vi "PH_SHS_Analysis.check Cam Settings.vi"(0 "i ref in":refnum<vi>, 5 "error in":errorcluster) -> (14 "i ref out":refnum<vi>, 19 "error out":errorcluster)   [LabVIEW 2014, in "PH_SHS_Analysis.lvlib"]
doc: "This VI checks whether the current cam setting equels the cam settings of the calibration data file and indicates the result at the GUI."
uses:
  PH_SHS_Analysis.lvlib
  PH_Basics/PH_StatusHandler/PH_StatusHandler.Status.ctl
  PH_Basics/PH_Common/PH_Common.lvlib
  PH_Basics/PH_Img_BaseClass/PH_Img_BaseClass.lvlib
  PH_Basics/PH_StatusHandler/PH_StatusHandler.lvlib
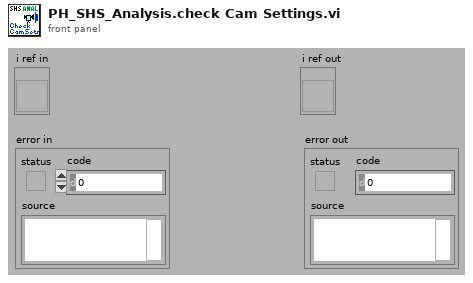
[diagram p1: front panel]
types:
  T1 = typedef "PH_StatusHandler.lvlib/PH_StatusHandler.Status.ctl" = i16
  T2 = typedef "PH_Img_BaseClass.lvlib/PH_Img_BaseClass.i attribute.ctl" = cluster{"GUI Refs":T3, "Timeout Image [ms]":i32, "Default Periodic Period [ms]":i32, "Camera":cluster{"Instancename":string, "Notifier":refnum<notifier>}, "Palette":T4, "Cam Settings":cluster{"Cam ID":string, "Gain":dbl, "Brightness":dbl, "Shutter":dbl, "Cam Info Failure":bool, "Mode":i32}}
  T3 = typedef "PH_Img_BaseClass.lvlib/PH_Img_BaseClass.GUI Refs.ctl" = cluster{"Timeout":refnum<vi>, "Image":refnum<vi>, "Palette":refnum<vi>, "Timeout Set":refnum<vi>}
  T4 = typedef "PH_Img_BaseClass.lvlib/PH_Img_BaseClass.Palette.ctl" = i32
  T5 = cluster{"Cam ID":string, "Gain":dbl, "Brightness":dbl, "Shutter":dbl, "Cam Info Failure":bool, "Mode":i32}
  T6 = typedef "PH_SHS_Analysis.lvlib/PH_SHS_Analysis.i attribute.ctl" = cluster{"GUI Refs":cluster{"Delete":refnum<vi>, "Global On":refnum<vi>, "Cam Source":refnum<vi>, "Calibration Data File":refnum<vi>, "Calibration status":refnum<vi>, "Show overlay":refnum<vi>, "SHS Device Config":refnum<vi>, "Result":refnum<vi>, "Consider Tilt":refnum<vi>, "Working Reference":refnum<vi>, "Remove Tilt":refnum<vi>, "Take Cali  Reference":refnum<vi>, "Publishing Data Status":refnum<vi>, "Calibration Data":refnum<vi>}, "Calibration":cluster{"Status":T1, "Data":T7, "File":path}, "Result":T12, "Image":T15, "SHS Device Config":T16, "Show Overlay":bool, "GradientZernikeMatrix":dbl[][], "Consider Tilt":bool, "Working Reference":T8, "Zernicke Service ID":i32, "PSDB Image":T15}
  T7 = typedef "PH_SHS_Analysis_Calibrator.lvlib/PH_SHS_Analysis_Calibrator.Analysis Calibration Data.ctl" = cluster{"Date":string, "Time":string, "Cam Settings":cluster{"Cam ID":string, "Gain":dbl, "Brightness":dbl, "Shutter":dbl, "Cam Error":bool, "Mode":i32}, "SHS Reference Result":T8, "Pixel Size":dbl, "MLA Pitch":dbl, "Method":enum16{"automatic", "manual"}, "Calibration Data calculated":bool, "No Problems at calculation?":bool, "error out":errorcluster}
  T8 = typedef "SHS_Common.lvlib/SHSReference.ctl" = cluster{"Reference":T9[][], "Lens Array Pitch [px]":dbl}
  T9 = typedef "SHS_Common.lvlib/ReferencePoint.ctl" = cluster{"Rect":T10, "Point":T11}
  T10 = typedef "SHS_Common.lvlib/Rectangle.ctl" = cluster{"Left":i32, "Top":i32, "Right":i32, "Bottom":i32}
  T11 = typedef "SHS_Common.lvlib/Point.ctl" = cluster{"x":dbl, "y":dbl, "valid?":bool, "weight":dbl}
  T12 = typedef "PH_SHS_Analysis.lvlib/PH_SHS_Analysis.Result.ctl" = cluster{"Time Stamp":timestamp, "Zernike Coefficients":T13, "PtV [lambda]":dbl, "Shifts":T14, "Measurement Quality":cluster{dbl, dbl, dbl}, "Measurement valid?":bool}
  T13 = typedef "PH_SHS_Analysis.lvlib/PH_SHS_Analysis.Zernike Coefficients.ctl" = cluster{"Tilt x":dbl, "Tilt y":dbl, "Defocus":dbl, "Astig 0°":dbl, "Astig 45°":dbl, "Coma x":dbl, "Coma y":dbl, "Spherical":dbl, "Trefoil 0°":dbl, "Trefoil 30°":dbl, "2nd Astig 0°":dbl, "2nd Astig 45°":dbl, "2nd Coma x":dbl, "2nd Coma y":dbl, "2nd Spherical":dbl}
  T14 = typedef "SHS_Common.lvlib/Shifts.ctl" = T11[][]
  T15 = typedef "IMAQ Image.ctl" = refnum<image>
  T16 = typedef "SHS_Analysis.lvlib/SHS_DeviceConfig.ctl" = cluster{"focal length [m]":dbl, "pixel size [m/px]":dbl, "wavelength [m]":dbl}
  T17 = cluster{"Cam ID":string, "Gain":dbl, "Brightness":dbl, "Shutter":dbl, "Cam Error":bool, "Mode":i32}
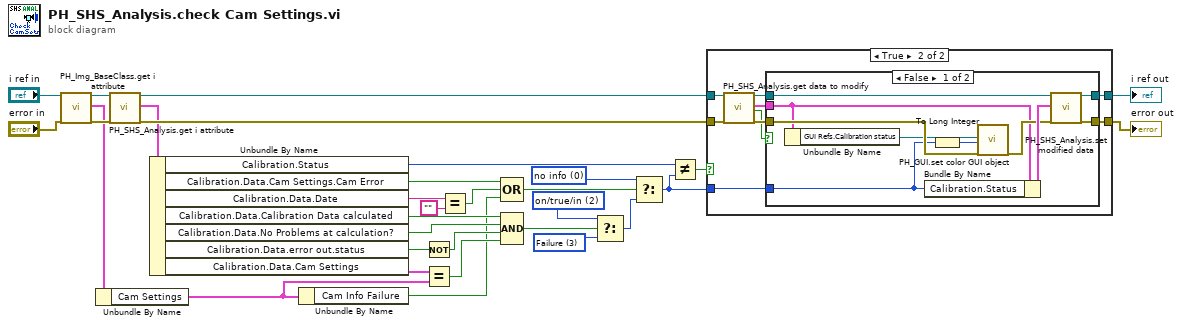
[diagram p0: block diagram]
diagram:
  w14 = T1 3 items=["no info", "off/false/out", "on/true/in", "Failure", "Alarm", "Status 1", "Status 2", "Status 3"] ("Calibration.Status")
  w15 = T1 2 items=["no info", "off/false/out", "on/true/in", "Failure", "Alarm", "Status 1", "Status 2", "Status 3"] ("Calibration.Status")
  w20 = T1 0 items=["no info", "off/false/out", "on/true/in", "Failure", "Alarm", "Status 1", "Status 2", "Status 3"] ("Calibration.Status")
  n1 = call "PH_Img_BaseClass.get i attribute.vi"("i ref in"="i ref in", "error in (no error)"="error in") -> ("i ref out"=w4:refnum<vi>, "i attribute"=w3:T2, "error out"=w6:errorcluster)  [unwired: 15 in]
  n2 = Unbundle By Name(w3) -> ("Cam Settings"=w2:T5)
  n3 = call "PH_SHS_Analysis.get i attribute.vi"("i ref in"=w4, "error in (no error)"=w6) -> ("i ref out"=w29:refnum<vi>, "i attribute"=w28:T6, "error out"=w30:errorcluster)  [unwired: 15 in]
  n4 = Unbundle By Name(w28) -> ("Calibration.Status"=w10:T1, "Calibration.Data.Cam Settings.Cam Error"=w27:bool, "Calibration.Data.Date"=w23:string, "Calibration.Data.Calibration Data calculated"=w19:bool, "Calibration.Data.No Problems at calculation?"=w18:bool, "Calibration.Data.error out.status"=w17:bool, "Calibration.Data.Cam Settings"=w12:T17)
  n5 = Unbundle By Name(w2) -> ("Cam Info Failure"=w1:bool)
  n6 = Not(x=w17) -> (.not. x?=w7:bool)
  n7 = Equal?(x=w12, y=w2) -> (x = y?=w11:bool)
  n8 = Equal?(x=w23, y="") -> (x = y?=w21:bool)
  n9 = Compound Arithmetic op=OR(w27, w21, w1) -> (w26:bool)
  n10 = Compound Arithmetic op=AND(w19, w18, w7, w11) -> (w16:bool)
  n11 = Select(t=w15, s=w16, f=w14) -> (s? t:f=w13:T1)
  n12 = Select(t=w20, s=w26, f=w13) -> (s? t:f=w9:T1)
  n13 = Not Equal?(x=w10, y=w9) -> (x != y?=w8:bool)
  n14 = case shown="True" w8 {
    tunnel: w30 -> [w32 w41]
    tunnel: w29 -> [w33 w40]
    tunnel: [w32 w39] -> w25
    tunnel: [w33 w37] -> w24
    tunnel: w9 -> [_ w34]
    frame False {
    }
    frame True {
      n15 = call "PH_SHS_Analysis.get data to modify.vi"("i ref in"=w40, "error in (no error)"=w41) -> ("i ref out"=w38:refnum<vi>, "i attribute"=w35:T6, "timed out"=w36:bool, "error out"=w42:errorcluster)  [unwired: 14 in]
      n16 = case shown="False" w36 {
        tunnel: w42 -> [w48 w53]
        tunnel: [w52 w53] -> w39
        tunnel: w38 -> [w51 w54]
        tunnel: [w50 w54] -> w37
        tunnel: w35 -> [w46 _]
        tunnel: w34 -> [w44 _]
        frame False {
          n17 = Unbundle By Name(w46) -> ("GUI Refs.Calibration status"=w45:refnum<vi>)
          n18 = Bundle By Name(cluster=w46, "Calibration.Status"=w44) -> (w49:T6)
          n19 = To Long Integer(number=w44) -> (32bit integer=w43:i32)
          n20 = call "PH_GUI.set color GUI object.vi"("GUI object Ref"=w45, "State"=w43, "error in (no error)"=w48) -> ("error out"=w47:errorcluster)  [unwired: 16 in]
          n21 = call "PH_SHS_Analysis.set modified data.vi"("i ref in"=w51, "i attribute"=w49, "error in (no error)"=w47) -> ("i ref out"=w50:refnum<vi>, "error out"=w52:errorcluster)  [unwired: 15 in]
        }
        frame True {
        }
      }
    }
  }
  "i ref out" <- w24
  "error out" <- w25
